vi "Test_PublishString_SubBeforePub_OK.vi"(8 "error in (no error)":errorcluster, 11 "TestMediator In":refnum<class "TestMediationSemantics.lvclass">) -> (0 "error out":errorcluster, 3 "TestMediator Out":refnum<class "TestMediationSemantics.lvclass">)   [LabVIEW 2020, in "TestMediationSemantics.lvclass"]
uses:
  TestMediationSemantics.lvclass
  TestMediationSemantics.lvclass/TestMediationSemantics.ctl
  Source/Mediator/Mediator/Mediator.lvclass
  <vilib>/ActorFramework/Actor/Actor.lvclass
  Source/IMediator/IMediator Messages/Publish Msg/Publish Msg.lvclass
  Source/IMediator/IMediator Messages/Subscribe Msg/Subscribe Msg.lvclass
  Source/IMediator/SubscriptionRequest/SubscriptionRequest.lvclass
  Source/IMediator/ISubscriptionPolicy/ISubscriptionPolicy.lvclass
  <vilib>/ActorFramework/Stop Msg/Stop Msg.lvclass
  Source/SubscriptionPolicy/BasicSubscription/BasicSubscription.lvclass
  modules/composed-transport/Source/Concrete/QueueTransport/QueueTransport.lvclass
  Source/IMediator/PublishRequest/PublishRequest.lvclass
  C:/Git/mva-core/Source/IMediator/IMediator/IMediator.lvclass
  C:/Program Files (x86)/National Instruments/LabVIEW 2020/vi.lib/ActorFramework/Actor/Actor.lvclass
  C:/Git/mva-core/Source/Mediator/Mediator/Mediator.lvclass
  C:/Git/mva-core/Source/IMediator/ISubscriptionPolicy/ISubscriptionPolicy.lvclass
  C:/Git/mva-core/Source/SubscriptionPolicy/BasicSubscription/BasicSubscription.lvclass
  C:/Git/mva-core/modules/composed-transport/Source/ITransport/ITransport.lvclass
  C:/Git/mva-core/modules/composed-transport/Source/Concrete/QueueTransport/QueueTransport.lvclass
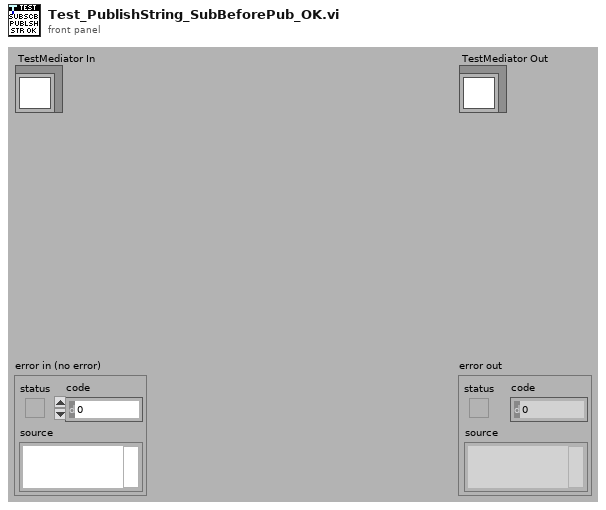
[diagram p1: front panel]
types:
  T1 = typedef "IMediator.lvlib/ISubscriptionPolicy.lvclass/ISubscriptionPolicy Reference.ctl" = refnum<data-value>
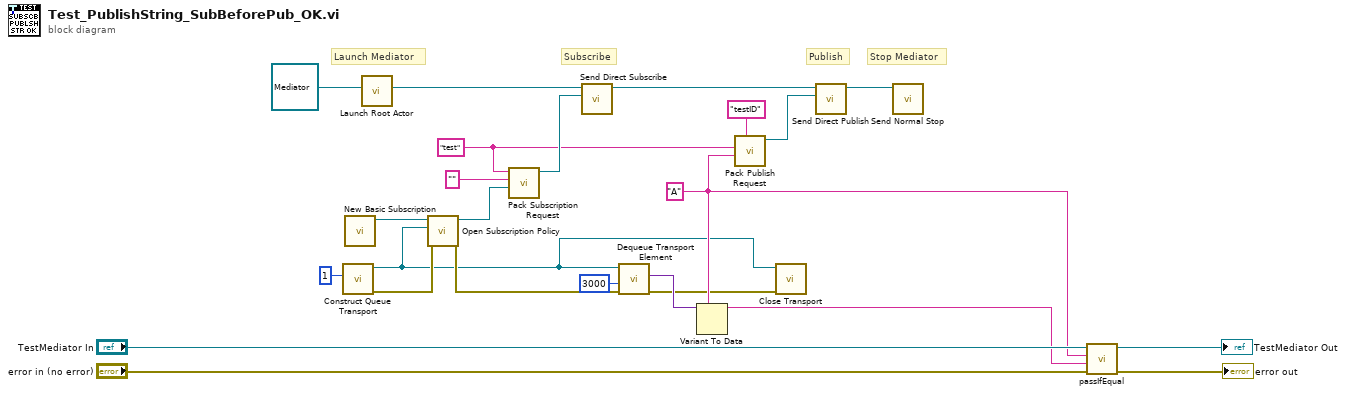
[diagram p0: block diagram]
diagram:
  w4 = "test" ("Datum Name")
  w3 = "A"
  # "Launch Mediator"
  # "Stop Mediator"
  # "Subscribe"
  # "Publish"
  n1 = call "Construct Queue Transport.vi"("Max Queue Size (-1)"=1) -> ("error out"=w15:errorcluster, "QueueTransport"=w2:refnum<class "QueueTransport.lvclass">)  [unwired: 9 in]
  n2 = call "New Basic Subscription.vi"() -> ("BasicSubscription Out"=w11:refnum<class "BasicSubscription.lvclass">)  [unwired: 11 in]
  n3 = call <vilib>:"Launch Root Actor.vi"("Actor"=refnum<class "Mediator.lvclass"> refnum ("Mediator.lvlib:Mediator.lvclass")) -> ("Actor's Enqueuer"=w8:refnum<class "Message Enqueuer.lvclass">)  [unwired: 9 in, 1 out]
  n4 = call "Open Subscription Policy.vi"("error in (no error)"=w15, "Transport"=w2, "SubscriptionPolicy"=w11) -> ("error out"=w14:errorcluster, "Subscription Policy"=w7:T1)  [unwired: 7 in]
  n5 = call "Pack Subscription Request.vi"("Subscription Policy"=w7, "Type"="", "Datum Name"=w4) -> ("SubscriptionRequest"=w19:refnum<class "SubscriptionRequest.lvclass">)  [unwired: 7 in, 1 out]
  n6 = call "Send Direct Subscribe.vi"("Subscription Request"=w19, "Message Enqueuer"=w8) -> ("Message Enqueuer out"=w10:refnum<class "Message Enqueuer.lvclass">)  [unwired: 8 in, 1 out]
  n7 = call "Dequeue Transport Element.vi"("error in (no error)"=w14, "Timeout In ms (-1)"=3000, "QueueTransport"=w2) -> ("error out"=w1:errorcluster, "Data"=w13:variant)  [unwired: 5 in, 2 out]
  n8 = Variant To Data(type=w3, Variant=w13) -> (data=w12:string)  [unwired: 1 in, 1 out]
  n9 = call "Pack Publish Request.vi"("Publisher ID"="testID", "Value"=w3, "Datum Name"=w4) -> ("PublishRequest Out"=w5:refnum<class "PublishRequest.lvclass">)  [unwired: 7 in, 1 out]
  n10 = call-dynamic "Close Transport.vi"("error in (no error)"=w1, "QueueTransport"=w2) -> ()  [unwired: 9 in, 1 out]
  n11 = call "Send Direct Publish.vi"("PublishRequest"=w5, "Mediator Enqueuer"=w10) -> ("Mediator Enqueuer out"=w9:refnum<class "Message Enqueuer.lvclass">)  [unwired: 8 in, 1 out]
  n12 = call <vilib>:"Send Normal Stop.vi"("Message Enqueuer"=w9) -> ()  [unwired: 10 in, 1 out]
  n13 = call-dynamic "passIfEqual.vi"("error in (no error)"="error in (no error)", "y"=w12, "x"=w3, "TestCase in"="TestMediator In") -> ("error out"=→"error out":errorcluster, "TestCase out"=→"TestMediator Out":refnum<class "TestMediationSemantics.lvclass">)  [unwired: 6 in]
